vi "Solution_Lab1.vi"() -> ()   [LabVIEW 2011]
uses:
  <vilib>/measure/maspectr.llb/FFT Spectrum (Mag-Phase) for 1 Chan.vi
  <vilib>/measure/NI_MABase.lvlib
  <vilib>/measure/NI_MAPro.lvlib
  <vilib>/ptbypt/NI_PtbyPt.lvlib
panel:
  in  "sample length":i32=1000
  out "Modulation Freq":dbl
  out "Baseband Freq":cluster{"f0":dbl, "df":dbl, "magnitude":dbl[]}(graph)
  out "AM":dbl
  out "Baseband":dbl
  out "Ratio: Base/AM":dbl
  out "Baseband Time":waveform(dbl)(graph)
  out "AM Freq":cluster{"f0":dbl, "df":dbl, "magnitude":dbl[]}(graph)
  in  "Modulation Index":dbl(slide)=1.0 scale=0.0..1.0
  in  "Modullation Freq":dbl(slide)=10.0 scale=0.0..1000.0
  in  "Carrier Freq":dbl(knob)=10.0 scale=0.0..500000.0
  out "AM Time":waveform(dbl)(graph)
  in  "stop":bool
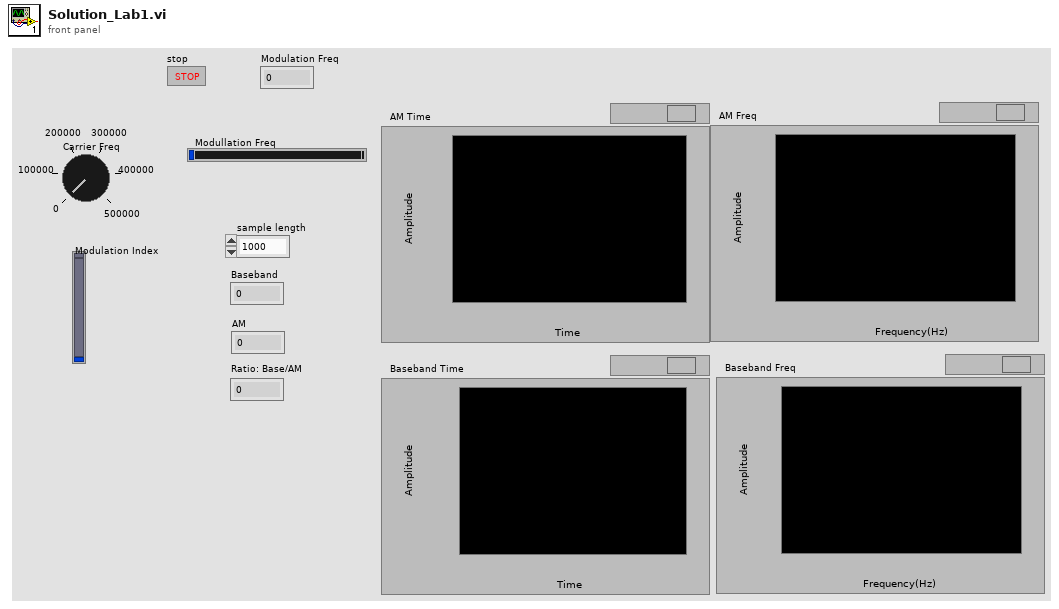
[diagram p1: front panel]
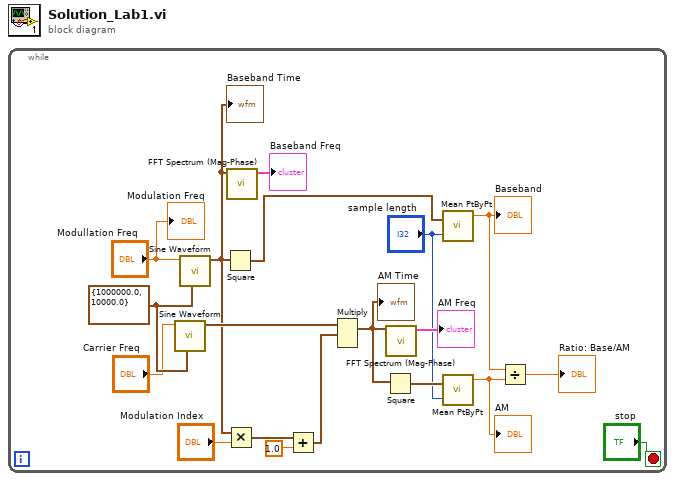
[diagram p0: block diagram]
diagram:
  n1 = while {
    stop <- "stop" stop-if-true
    w18 = cluster{"Fs":dbl, "#s":dbl} {"Fs"=1000000.0, "#s"=10000.0} ("sampling info")
    n2 = call <vilib>:"Sine Waveform.vi"("sampling info"=w18, "frequency"="Carrier Freq") -> ("signal out"=w12:waveform(dbl))  [unwired: 8 in, 1 out]
    n3 = call <vilib>:"Sine Waveform.vi"("sampling info"=w18, "frequency"="Modullation Freq") -> ("signal out"=w8:waveform(dbl))  [unwired: 8 in, 1 out]
    "Baseband Time" <- w8
    n4 = Square(x=w8) -> (x^2=w1:waveform(dbl))
    n5 = Multiply(x=w8, y="Modulation Index") -> (x*y=w9:waveform(dbl))
    n6 = call-poly <vilib>:"FFT Spectrum (Mag-Phase).vi"("time signal"=w8) -> ("magnitude"=→"Baseband Freq":cluster{"f0":dbl, "df":dbl, "magnitude":dbl[]})  [unwired: 6 in, 4 out]
    n7 = Add(x=w9, y=1.0) -> (x+y=w11:waveform(dbl))
    n8 = Multiply(1:w11, 2:w12) -> (0:w13:waveform(dbl))  [unwired: 1 in, 1 out]
    "AM Time" <- w13
    n9 = Square(x=w13) -> (x^2=w6:waveform(dbl))
    n10 = call-poly <vilib>:"FFT Spectrum (Mag-Phase).vi"("time signal"=w13) -> ("magnitude"=→"AM Freq":cluster{"f0":dbl, "df":dbl, "magnitude":dbl[]})  [unwired: 6 in, 4 out]
    n11 = call <vilib>:"Mean PtByPt.vi"("x"=w1, "sample length"="sample length") -> ("mean"=w4:dbl)  [unwired: 2 in, 1 out]
    "Baseband" <- w4
    n12 = call <vilib>:"Mean PtByPt.vi"("x"=w6, "sample length"="sample length") -> ("mean"=w5:dbl)  [unwired: 2 in, 1 out]
    "AM" <- w5
    n13 = Divide(x=w4, y=w5) -> (x/y=→"Ratio: Base/AM":dbl)
    "Modulation Freq" <- "Modullation Freq"
  }
